vi "main_ctrl.vi"(8 "error in":errorcluster) -> (0 "error out":errorcluster)   [LabVIEW 2011]
uses:
  fg_typedef.ctl
  vision enable.ctl
  vision data.ctl
  singleUseSubstate.ctl
  subStates.ctl
  <vilib>/Rock Robotics/WPI/Solenoid/WPI_SolenoidValue.ctl
  <vilib>/Rock Robotics/WPI/Compressor/WPI_CompressorGetSetRefNum.vi
  <vilib>/Rock Robotics/WPI/Solenoid/WPI_SolenoidGetEnum.vi
  <vilib>/Rock Robotics/WPI/Solenoid/WPI_SolenoidSetEnum.vi
  <vilib>/addons/control/pid/pid.llb/PID Control Input Filter (DBL).vi
  <vilib>/addons/control/pid/NI_PID_pid.lvlib
  <vilib>/Rock Robotics/WPI/RobotDrive/WPI_RobotDriveArcadeDrive_Standard(NoSaturation).vi
panel:
  out "Vision SPI":u32
  out "Vision IPS":dbl
  out "IPS":dbl
  out "SPI":u32
  # "MAIN CONTROL"
  # "holds robot control code - dual parallel state machine"
  # "SPI: milliseconds per iteration\nIPS: iterations per second"
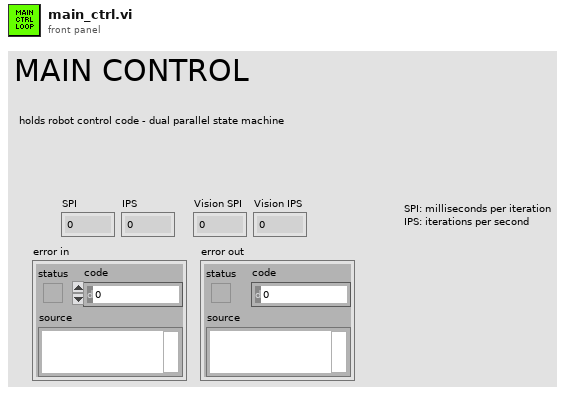
[diagram p1: front panel]
types:
  T1 = typedef "vision data.ctl" = cluster{"x":dbl, "y":dbl, "area":dbl, "width":dbl, "height":dbl}
  T2 = typedef "vision enable.ctl" = enum16{"Enable", "Disable", "Stop"}
  T3 = typedef "fg_typedef.ctl" = enum16{"Get", "Set"}
  T4 = typedef "WPI_CameraDevRef.ctl" = cluster{"Camera Address":string, "CameraStatus":errorcluster, "Acquire Image Notifier":refnum<notifier>}
  T5 = typedef "WPI_CompressorDevRef.ctl" = cluster{"DevStatus":errorcluster, "DigitalInputDevRef":T6, "RelayDevRef":T9}
  T6 = typedef "WPI_DigitalInputDevRef.ctl" = cluster{"DevStatus":errorcluster, "DIO Channel":T7, "Digital Module":T8}
  T7 = typedef "FPGA_DIOChannel.ctl" = enum8{"DIO 1", "DIO 2", "DIO 3", "DIO 4", "DIO 5", "DIO 6", "DIO 7", "DIO 8", "DIO 9", "DIO 10", "DIO 11", "DIO 12", "DIO 13", "DIO 14", "Invalid"}
  T8 = typedef "FPGA_TypedefDigitalModule.ctl" = enum16{"Digital Module 1", "Digital Module 2"}
  T9 = typedef "WPI_RelayDevRef.ctl" = cluster{"DevStatus":errorcluster, "Relay Channel":T10, "Digital Module":T8, "Relay Direction":T11}
  T10 = typedef "FPGA_DIORelayChannel.ctl" = enum8{"Relay 1", "Relay 2", "Relay 3", "Relay 4", "Relay 5", "Relay 6", "Relay 7", "Relay 8", "Invalid"}
  T11 = typedef "WPI_RelayDirection.ctl" = enum16{"Both directions", "Forward only", "Reverse only"}
  T12 = typedef "IMAQ Image.ctl" = refnum<image>
  T13 = typedef "WPI_SolenoidValue.ctl" = enum16{"Off", "On", "Forward", "Reverse"}
  T14 = typedef "singleUseSubstate.ctl" = enum16{"null", "wait", "shift", "shift high", "shift low", "bridge down", "bridge up", "extender in", "extender out", "extender toggle", "end"}
  T15 = typedef "WPI_DriverStationDerivedRobotMode.ctl" = enum16{"Init", "Execute", "Stop"}
  T16 = typedef "WPI_DriverStationRobotMode.ctl" = enum16{"Autonomous Disabled", "Autonomous Enabled", "Teleop Disabled", "Teleop Enabled", "Timeout", "Finish"}
  T17 = typedef "subStates.ctl" = enum16{"null", "wait", "driver control", "auto", "manual override", "autoDrive", "hold position", "rotate", "end"}
  T18 = typedef "WPI_SolenoidDevRef.ctl" = cluster{"DevStatus":errorcluster, "Solenoid Module":T19, "Forward Solenoid Channel":T20, "Reverse Solenoid Channel":T20}
  T19 = typedef "FPGA_TypedefSolenoidModule.ctl" = enum16{"Solenoid Module 1", "Solenoid Module 2"}
  T20 = typedef "WPI_SolenoidChannel.ctl" = enum8{"Solenoid 1", "Solenoid 2", "Solenoid 3", "Solenoid 4", "Solenoid 5", "Solenoid 6", "Solenoid 7", "Solenoid 8", "Invalid"}
  T21 = typedef "WPI_RobotDriveDevRef.ctl" = cluster{"DevStatus":errorcluster, "Motors[]":T22[], "Square Inputs":bool, "Max Output":dbl, "Isochronous":bool}
  T22 = typedef "WPI_MotorControlDeviceRef.ctl" = cluster{"DeviceStatus":errorcluster, "Type":enum16{"PWM", "CAN"}, "PWM":cluster{"Digital Module":T8, "PWM Channel":T23, "DeadBand":T24}, "CAN":cluster{"Device Number":u8, "Control Mode":T25, "Semaphore":T26, "Max Vout":dbl}, "Invert":bool, "TransformRef":T27, "InvTransformRef":T27}
  T23 = typedef "FPGA_DIOPWMChannel.ctl" = enum8{"PWM 1", "PWM 2", "PWM 3", "PWM 4", "PWM 5", "PWM 6", "PWM 7", "PWM 8", "PWM 9", "PWM 10", "Invalid"}
  T24 = typedef "WPI_PWMDeadband.ctl" = cluster{"Name":string, "maxPositivePwm":i32, "minPositivePwm":i32, "centerPwm":i32, "maxNegativePwm":i32, "minNegativePwm":i32, "angularRange":u16}
  T25 = typedef "WPI_CANJaguar_ControlMode.ctl" = enum8{"Percent VBus", "Current", "Speed", "Position", "Voltage"}
  T26 = typedef "Semaphore RefNum" = refnum<k1>
  T27 = typedef "WPI_PWMTransform_ConPane.ctl" = refnum<vi>
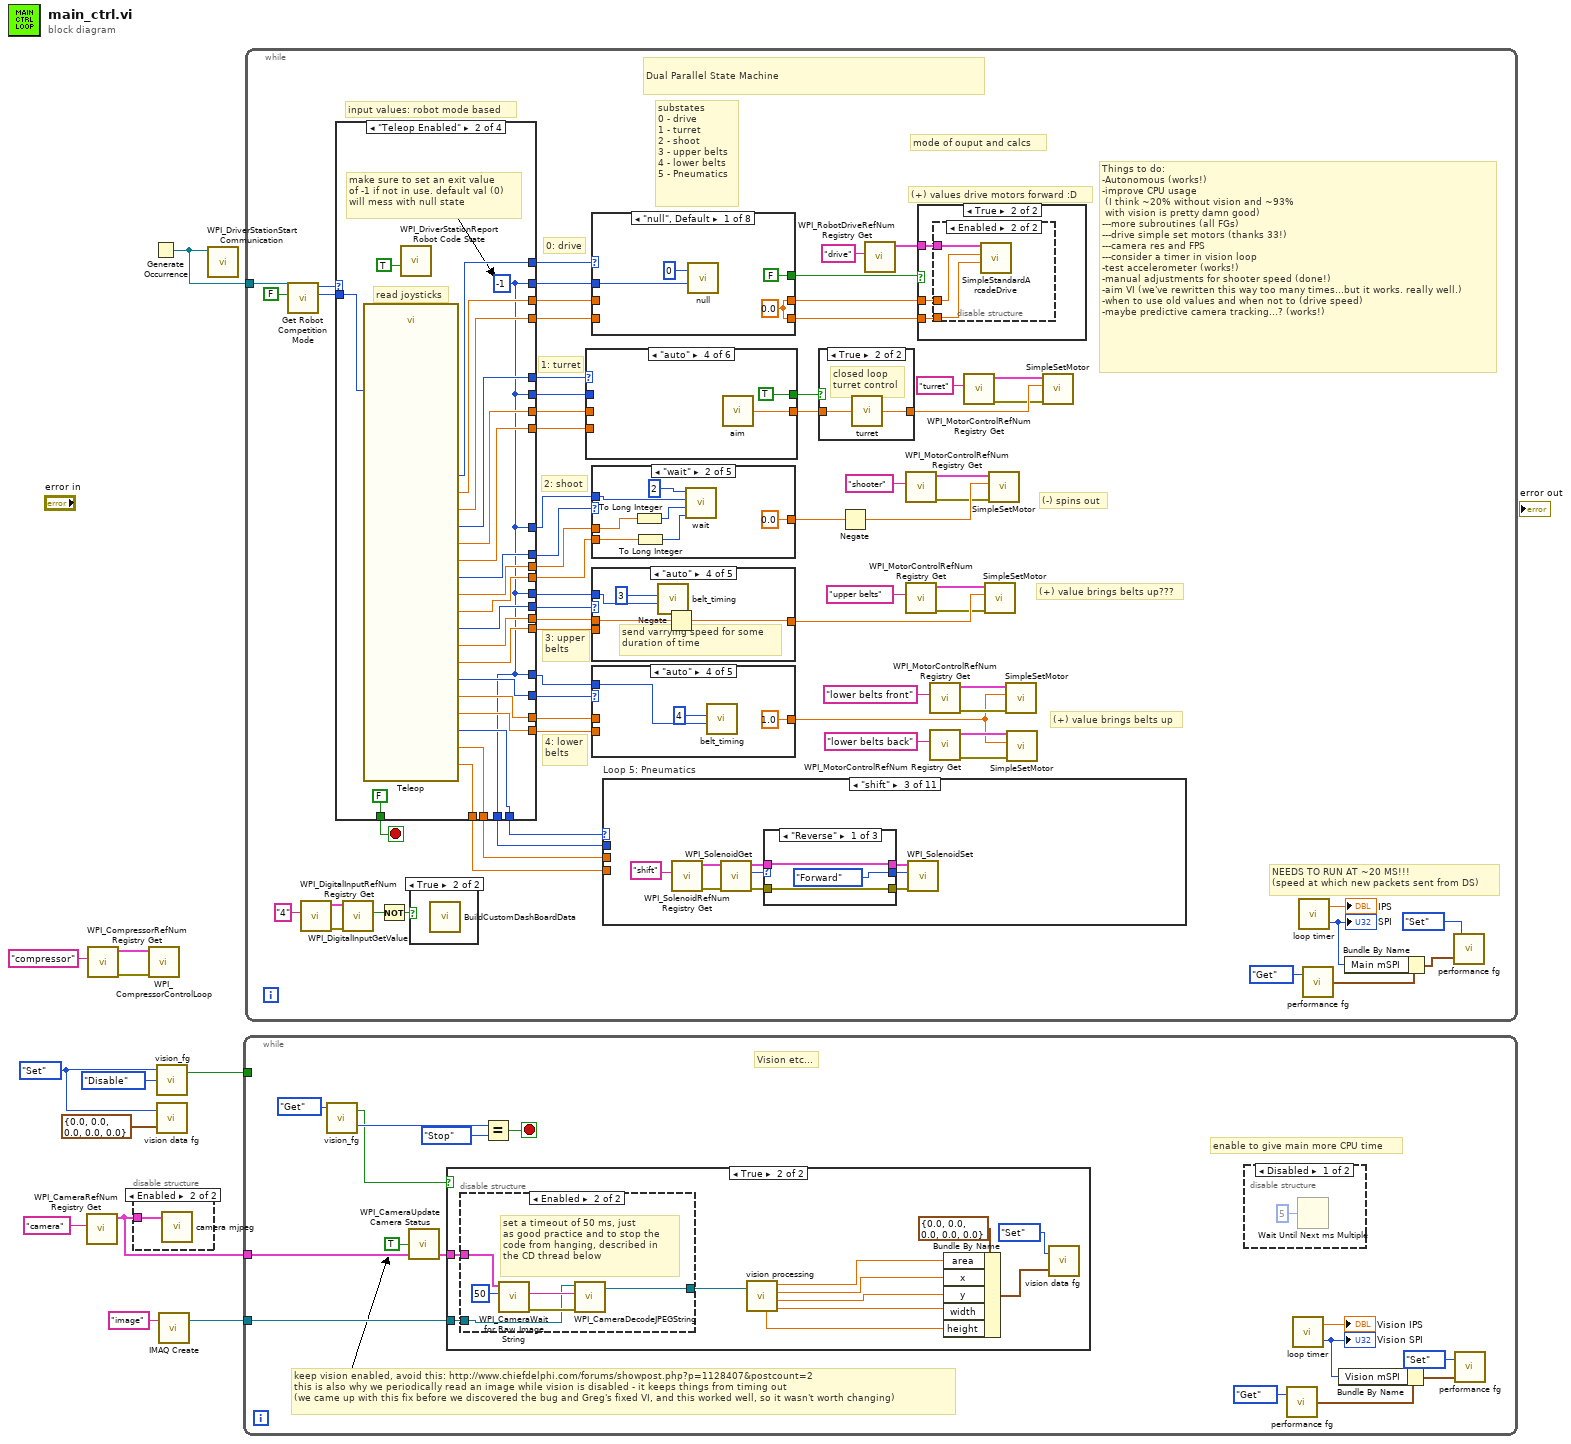
[diagram p0: block diagram]
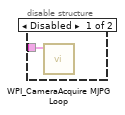
[diagram p2: hidden frame]
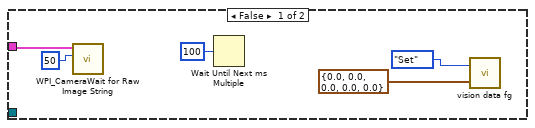
[diagram p4: hidden frame]
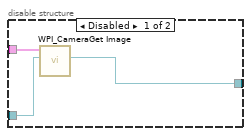
[diagram p5: hidden frame]
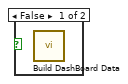
[diagram p6: hidden frame]
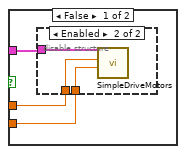
[diagram p8: hidden frame]
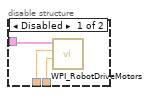
[diagram p9: hidden frame]
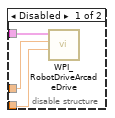
[diagram p10: hidden frame]
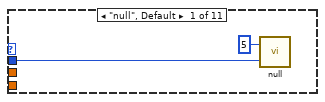
[diagram p11: hidden frame]
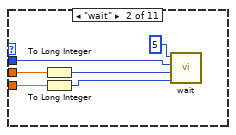
[diagram p12: hidden frame]
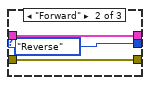
[diagram p13: hidden frame]
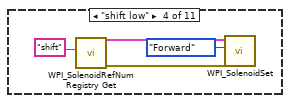
[diagram p15: hidden frame]
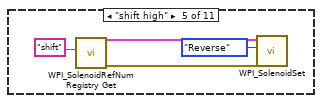
[diagram p16: hidden frame]
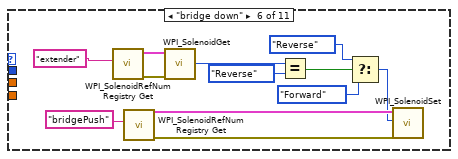
[diagram p17: hidden frame]
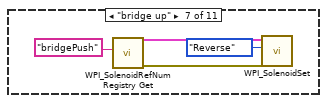
[diagram p18: hidden frame]
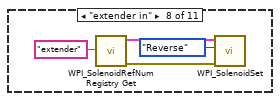
[diagram p19: hidden frame]
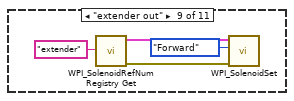
[diagram p20: hidden frame]
diagram:
  w9 = fg_typedef."Set" ("Enum")
  n1 = call <vilib>:"WPI_CameraRefNum Registry Get.vi"("refnum name"="camera") -> ("CameraDevRef"=w2:T4)  [unwired: 9 in, 1 out]
  n2 = call <vilib>:"WPI_CompressorRefNum Registry Get.vi"("refnum name"="compressor") -> ("error out"=w5:errorcluster, "CompressorDevRef"=w6:T5)  [unwired: 9 in]
  n3 = disable-structure shown="Enabled" {
    disable-tunnel: w2 -> [w13 w14]
    frame Disabled {
      n4 = call <vilib>:"WPI_CameraAcquire MJPG Loop.vi"("CameraDevRef"=w13) -> ()  [unwired: 11 in]
    }
    frame Enabled {
      n5 = call "camera mjpeg.vi"("CameraDevRef"=w14) -> ()  [unwired: 11 in]
    }
  }
  n6 = call <vilib>:"WPI_CompressorControlLoop.vi"("error in (no error)"=w5, "CompressorDevRef"=w6) -> ()  [unwired: 10 in]
  n7 = Generate Occurrence() -> (w12:refnum<k4>)
  n8 = call "vision_fg.vi"("Action"=vision_enable."Disable", "Menu"=w9) -> ("Enabled?"=w10:bool)  [unwired: 1 in, 1 out]
  n9 = call "vision data fg.vi"("Input"=T1 {"x"=0.0, "y"=0.0, "area"=0.0, "width"=0.0, "height"=0.0} ("Cluster"), "Menu"=w9) -> ()  [unwired: 1 out]
  n10 = call "IMAQ Create"("Image Name"="image") -> ("New Image"=w11:T12)  [unwired: 4 in, 1 out]
  n11 = call <vilib>:"WPI_DriverStationStart Communication.vi"("occurrence"=w12) -> ()  [unwired: 11 out]
  n12 = while {
    tunnel: w11 -> [w28]
    tunnel: w2 -> [w27]
    tunnel: w10 -> [_]
    stop <- w29 stop-if-true
    # "keep vision enabled, avoid this: http://www.chiefdelphi.com/forums/showpost.php?p=1128407&postcount=2\nthis is also why we periodically read an image while vision is disabled - it keeps things from timing out\n(we came up with this fix before we discovered the bug and Greg's fixed VI, and this worked well, so it wasn't worth changing)"
    # "enable to give main more CPU time"
    # "Vision etc..."
    n13 = call "vision_fg.vi"("Menu"=fg_typedef."Get" ("Enum")) -> ("State Out"=w23:T2, "Enabled?"=w15:bool)  [unwired: 2 in]
    n14 = call <vilib>:"WPI_CameraUpdate Camera Status.vi"("CameraDevRef In"=w27, "Enable Vision"=TRUE) -> ("CameraDevRef Out"=w26:T4)  [unwired: 3 in]
    n15 = case shown="True" w15 {
      tunnel: w28 -> [_ w46]
      tunnel: w26 -> [w33 w45]
      frame False {
        n16 = call <vilib>:"WPI_CameraWait for Raw Image String.vi"("Timeout in ms (-1)"=50, "CameraDevRef"=w33) -> ()  [unwired: 3 in, 7 out]
        n17 = Wait Until Next ms Multiple(millisecond multiple=u32 100) -> ()  [unwired: 1 out]
        n18 = call "vision data fg.vi"("Input"=T1 {"x"=0.0, "y"=0.0, "area"=0.0, "width"=0.0, "height"=0.0} ("Cluster"), "Menu"=fg_typedef."Set" ("Enum")) -> ()  [unwired: 1 out]
      }
      frame True {
        n19 = disable-structure shown="Enabled" {
          disable-tunnel: w46 -> [w49 w51]
          disable-tunnel: w45 -> [w48 w53]
          disable-tunnel: [w47 w50] -> w42
          frame Disabled {
            n20 = call <vilib>:"WPI_CameraGet Image.vi"("Image"=w49, "CameraDevRef"=w48) -> ("Image Out"=w47:T12)  [unwired: 7 in, 2 out]
          }
          frame Enabled {
            # "set a timeout of 50 ms, just\nas good practice and to stop the \ncode from hanging, described in \nthe CD thread below"
            n21 = call <vilib>:"WPI_CameraWait for Raw Image String.vi"("Timeout in ms (-1)"=50, "CameraDevRef"=w53) -> ("error out"=w55:errorcluster, "String"=w54:string)  [unwired: 3 in, 5 out]
            n22 = call <vilib>:"WPI_CameraDecodeJPEGString.vi"("error in"=w55, "Compressed Image"=w54, "Image In"=w51) -> ("Image Out"=w50:T12)  [unwired: 4 out]
          }
        }
        n23 = call "vision processing.vi"("Image In"=w42) -> ("height"=w39:dbl, "area"=w38:dbl, "x"=w37:dbl, "y"=w36:dbl, "width"=w40:dbl)  [unwired: 1 in, 1 out]
        n24 = Bundle By Name(cluster=T1 {"x"=0.0, "y"=0.0, "area"=0.0, "width"=0.0, "height"=0.0} ("Cluster"), "area"=w38, "x"=w37, "y"=w36, "width"=w40, "height"=w39) -> (w41:T1)
        n25 = call "vision data fg.vi"("Input"=w41, "Menu"=fg_typedef."Set" ("Enum")) -> ()  [unwired: 1 out]
      }
    }
    n26 = Equal?(x=w23, y=vision_enable."Stop") -> (x = y?=w29:bool)
    n27 = disable-structure shown="Disabled" {
      frame Disabled {
        n28 = Wait Until Next ms Multiple(millisecond multiple=u32 5) -> ()  [unwired: 1 out]
      }
      frame Enabled {
      }
    }
    n29 = call "performance fg.vi"("Menu"=fg_typedef."Get") -> ("Output"=w18:cluster{"Vision mSPI":u32, "Main mSPI":u32})  [unwired: 1 in]
    n30 = call "loop timer.vi"() -> ("IPS"=→"Vision IPS":dbl, "SPI"=w20:u32)  [unwired: 1 in]
    "Vision SPI" <- w20
    n31 = Bundle By Name(cluster=w18, "Vision mSPI"=w20) -> (w17:cluster{"Vision mSPI":u32, "Main mSPI":u32})
    n32 = call "performance fg.vi"("Input"=w17, "Menu"=fg_typedef."Set") -> ()  [unwired: 1 out]
  }
  n33 = while {
    tunnel: w12 -> [w121]
    stop <- w96 stop-if-true
    # "input values: robot mode based"
    # "Things to do:\n-Autonomous (works!)\n-improve CPU usage\n (I think ~20% without vision and ~93% \n with vision is pretty damn good)\n---more subroutines (all FGs)\n---drive simple set motors (thanks 33!)\n---camera res and FPS\n---consider a timer in vision loop\n-test accelerometer (works!)\n-manual adjustments for shooter speed (done!)\n-aim VI (we've rewritten this way too many times...but it works. really well.)\n-when to use old values and when not to (drive speed)\n-maybe predictive camera tracking...? (works!)"
    # "(-) spins out"
    # "(+) value brings belts up"
    # "(+) values drive motors forward :D"
    # "(+) value brings belts up???"
    # "mode of ouput and calcs"
    # "4: lower\nbelts"
    # "3: upper\nbelts"
    # "2: shoot"
    # "1: turret"
    # "0: drive"
    # "substates\n0 - drive\n1 - turret\n2 - shoot\n3 - upper belts\n4 - lower belts\n5 - Pneumatics"
    # "NEEDS TO RUN AT ~20 MS!!!\n(speed at which new packets sent from DS)"
    # "Dual Parallel State Machine"
    n34 = call "Get Robot Competition Mode.vi"("Finish"=FALSE, "DS Occurrence"=w121) -> ("Call Context"=w110:T15, "Robot Mode"=w120:T16)  [unwired: 6 in, 2 out]
    n35 = call <vilib>:"WPI_DigitalInputRefNum Registry Get.vi"("refnum name"="4") -> ("error out"=w73:errorcluster, "DigitalInputDevRef"=w72:T6)  [unwired: 9 in]
    n36 = case shown="\"Teleop Enabled\"" w120 {
      tunnel: [w342 w364 w368 w380] -> w82
      tunnel: [w341 w361 w368 w380] -> w119
      tunnel: [w340 w345 w366 _] -> w118
      tunnel: [w339 w363 _ _] -> w117
      tunnel: [w338 w362 _ _] -> w116
      tunnel: [w337 w345 w366 _] -> w115
      tunnel: [w336 w359 _ _] -> w114
      tunnel: [w335 w358 _ _] -> w113
      tunnel: w110 -> [w334 w343 _ _]
      tunnel: [w333 w360 w368 w380] -> w107
      tunnel: [w332 w357 _ _] -> w106
      tunnel: [w331 w356 w368 w380] -> w105
      tunnel: [w327 w355 w368 w380] -> w104
      tunnel: [w330 w354 _ _] -> w103
      tunnel: [w326 w353 _ _] -> w102
      tunnel: [w329 w352 _ _] -> w100
      tunnel: [w325 w351 _ _] -> w99
      tunnel: [w324 w346 singleUseSubstate."null" ("SubState 5") singleUseSubstate."end" ("SubState 5")] -> w97
      tunnel: [FALSE FALSE FALSE TRUE] -> w96
      tunnel: [w328 w345 w366 _] -> w83
      tunnel: [w323 w345 w366 _] -> w88
      tunnel: [w322 w345 w366 _] -> w87
      tunnel: [w319 w349 _ _] -> w86
      tunnel: [w318 w348 _ _] -> w85
      tunnel: [w320 w345 w366 _] -> w84
      tunnel: [w317 w347 _ _] -> w80
      frame "Autonomous Enabled" {
        n37 = call "autoSM.vi"("Call Context"=w334) -> ("Loop 2 SubState"=w333:T17, "Loop 2 exit value"=w328:i32, "Loop 2 Value 2"=w317:dbl, "Loop 3 Value 1"=w330:dbl, "Loop 3 Value 2"=w329:dbl, "Loop 2 Value 1"=w332:dbl, "Loop 3 SubState"=w331:T17, "Loop 4 SubState"=w327:T17, "Loop 4 exit value"=w322:i32, "Loop 0 SubState"=w342:T17, "Loop 1 SubState"=w341:T17, "Loop 0 exit value"=w340:i32, "Loop 1 exit value"=w337:i32, "Loop 4 Value 2"=w325:dbl, "Loop 3 exit value"=w323:i32, "Loop 4 Value 1"=w326:dbl, "Pneumatics SubState"=w324:T14, "Loop 0 Value 1"=w339:dbl, "Loop 5 Exit Value"=w320:i32, "Loop 5 Value 2"=w318:dbl, "Loop 0 Value 2"=w338:dbl, "Loop 1 Value 1"=w336:dbl, "Loop 5 Value 1"=w319:dbl, "Loop 1 Value 2"=w335:dbl)  [unwired: 3 in]
        n38 = call <vilib>:"WPI_DriverStationReport Robot Code State.vi"("Autonomous"=TRUE) -> ()  [unwired: 10 in, 1 out]
      }
      frame "Teleop Enabled" {
        w345 = -1 ("Loop 0 exit value")
        # "make sure to set an exit value\nof -1 if not in use. default val (0) \nwill mess with null state"
        # "read joysticks"
        n39 = call "Teleop.vi"("Call Context"=w343) -> ("Loop 5 Value 1"=w349:dbl, "Loop 5 Value 2"=w348:dbl, "Loop 2 Value 2"=w347:dbl, "Loop 2 Value 1"=w357:dbl, "Loop 0 Value 1"=w363:dbl, "Loop 1 Value 2"=w358:dbl, "Loop 4 Value 2"=w351:dbl, "SubState 5"=w346:T14, "Loop 0 Value 2"=w362:dbl, "Loop 1 Value 1"=w359:dbl, "Loop 3 Value 2"=w352:dbl, "Loop 3 Value 1"=w354:dbl, "SubState 0"=w364:T17, "SubState 4"=w355:T17, "SubState 3"=w356:T17, "SubState 1"=w361:T17, "Loop 4 Value 1"=w353:dbl, "SubState 2"=w360:T17)  [unwired: 1 in]
        n40 = call <vilib>:"WPI_DriverStationReport Robot Code State.vi"("TeleOp"=TRUE) -> ()  [unwired: 10 in, 1 out]
      }
      frame "Autonomous Disabled", "Teleop Disabled", "Timeout" {
        w366 = -1 ("Loop 0 exit value")
        w368 = subStates."null" ("SubState 0")
        # "exit value of -1"
        # "set all loops to null"
        # "make sure to disable vision\nwe don't need it here"
        # "robot disabled, timeout"
        n41 = call "vision_fg.vi"("Action"=vision_enable."Disable", "Menu"=fg_typedef."Set") -> ()  [unwired: 1 in, 2 out]
        n42 = call <vilib>:"WPI_DriverStationReport Robot Code State.vi"("Disabled"=TRUE) -> ()  [unwired: 10 in, 1 out]
      }
      frame "Finish" {
        w380 = subStates."end"  # Stop All Loops
        # "stop the while loop"
        # "stop DS comms"
        # "stop compressor"
        # "stop vision loop"
        n43 = call <vilib>:"WPI_DriverStationStop Communication.vi"("StopCommunication"=TRUE) -> ()  [unwired: 10 in, 1 out]
        n44 = call <vilib>:"WPI_CompressorRefNum Registry Get.vi"("refnum name"="compressor") -> ("error out"=w374:errorcluster, "CompressorDevRef"=w373:T5)  [unwired: 9 in]
        n45 = call "vision_fg.vi"("Action"=vision_enable."Stop", "Menu"=fg_typedef."Set") -> ()  [unwired: 1 in, 2 out]
        n46 = call <vilib>:"WPI_CompressorClose.vi"("error in (no error)"=w374, "CompressorDevRef"=w373) -> ()  [unwired: 9 in, 1 out]
      }
    }
    n47 = call <vilib>:"WPI_DigitalInputGetValue.vi"("error in (no error)"=w73, "DigitalInputDevRef"=w72) -> ("Value"=w71:bool)  [unwired: 7 in, 2 out]
    n48 = Not(x=w71) -> (.not. x?=w70:bool)
    n49 = case shown="True" w70 {
      frame False {
        n50 = call "Build DashBoard Data.vi"() -> ()  [unwired: 12 in]
      }
      frame True {
        n51 = call "BuildCustomDashBoardData.vi"() -> ()  [unwired: 12 out]
      }
    }
    n52 = case shown="\"auto\"" w119 {
      tunnel: w115 -> [w255 w263 _ _ _ _]
      tunnel: w114 -> [_ w262 w266 _ _ w273]
      tunnel: w113 -> [_ w260 _ _ _ _]
      tunnel: [0.0 ("Loop 0 Value1") 0.0 ("Loop 1 Value1") w266 w269 0.0 ("Loop 0 Value1") w272] -> w101
      tunnel: [TRUE TRUE TRUE TRUE TRUE FALSE] -> w98
      frame "null", Default {
        n53 = call "null.vi"("Exit Loop ID"=w255, "This Loop ID"=1) -> ()  [unwired: 1 in]
      }
      frame "wait" {
        n54 = To Long Integer(number=w262) -> (32bit integer=w261:i32)
        n55 = To Long Integer(number=w260) -> (32bit integer=w259:i32)
        n56 = call "wait.vi"("State to wait for"=w259, "Waiting Loop ID"=w261, "time (ms)"=w263, "Current Loop ID"=1) -> ()  [unwired: 1 out]
      }
      frame "driver control" {
      }
      frame "auto" {
        n57 = call "aim.vi"() -> ("rate"=w269:dbl)  [unwired: 2 in]
      }
      frame "end" {
      }
      frame "manual override" {
        n58 = expression code="-x/4"(w273) -> (w272:dbl)
      }
    }
    n59 = case shown="\"null\", Default" w82 {
      tunnel: w118 -> [w275 w285 _ _ _ _ _ _]
      tunnel: w117 -> [_ w282 w290 w294 w298 w305 w310 _]
      tunnel: w116 -> [_ w281 w289 w293 w297 w304 w309 _]
      tunnel: [w278 w284 w288 w296 w300 w306 w312 w315] -> w112
      tunnel: [w278 w284 w287 w295 w299 w307 w311 w315] -> w111
      tunnel: [FALSE FALSE TRUE w292 FALSE ("Drive Type") FALSE ("Drive Type") FALSE ("Drive Type") FALSE] -> w109
      frame "null", Default {
        w278 = 0.0 ("Drive Value1")
        n60 = call "null.vi"("Exit Loop ID"=w275, "This Loop ID"=0) -> ()  [unwired: 1 in]
      }
      frame "wait" {
        w284 = 0.0 ("Drive Value1")
        # "wait on timer or parallel state"
        n61 = To Long Integer(number=w282) -> (32bit integer=w280:i32)
        n62 = To Long Integer(number=w281) -> (32bit integer=w279:i32)
        n63 = call "wait.vi"("State to wait for"=w279, "Waiting Loop ID"=w280, "time (ms)"=w285, "Current Loop ID"=0) -> ()  [unwired: 1 out]
      }
      frame "driver control" {
        n64 = Negate(x=w290) -> (-x=w288:dbl)
        n65 = Negate(x=w289) -> (-x=w287:dbl)
      }
      frame "auto" {
        n66 = call "balance.vi"("Joystick X"=w294, "Joystick Y"=w293) -> ("Drive Type"=w292:bool, "left"=w296:dbl, "right"=w295:dbl)
      }
      frame "autoDrive" {
        n67 = call "autoDrive.vi"("Rate"=w297, "Distance to Travel"=w298) -> ("right speed"=w299:dbl, "left speed"=w300:dbl)  [unwired: 1 in, 1 out]
      }
      frame "hold position" {
        n68 = Negate(x=w305) -> (-x=w303:dbl)
        n69 = Negate(x=w304) -> (-x=w302:dbl)
        n70 = call "closed drive.vi"("Y axis value"=w302, "X axis value"=w303) -> ("right"=w307:dbl, "left"=w306:dbl)
      }
      frame "rotate" {
        n71 = call "rotate.vi"("Angle"=w310, "Rate"=w309) -> ("left speed"=w312:dbl, "right speed"=w311:dbl)  [unwired: 1 out]
      }
      frame "end" {
        w315 = 0.0 ("Loop 0 Value1")
      }
    }
    n72 = case shown="\"wait\"" w107 {
      tunnel: w106 -> [_ w245 w249 _ _]
      tunnel: [0.0 ("Loop 2 Value 1") 0.0 ("Loop 2 Value 1") w248 w251 0.0 ("Loop 2 Value 1")] -> w81
      tunnel: w83 -> [w238 w244 _ _ _]
      tunnel: w80 -> [_ w241 _ _ _]
      frame "null", Default {
        n73 = call "null.vi"("Exit Loop ID"=w238, "This Loop ID"=2) -> ()  [unwired: 1 in]
      }
      frame "wait" {
        n74 = To Long Integer(number=w245) -> (32bit integer=w243:i32)
        n75 = To Long Integer(number=w241) -> (32bit integer=w242:i32)
        n76 = call "wait.vi"("State to wait for"=w242, "Waiting Loop ID"=w243, "time (ms)"=w244, "Current Loop ID"=2) -> ()  [unwired: 1 out]
      }
      frame "driver control", "manual override" {
        n77 = expression code="(-x +1) / 2" "can't drive shooter back"(w249) -> (w248:dbl)
      }
      frame "auto" {
        n78 = call "calc shooter speed.vi"() -> ("Speed"=w252:dbl)  [unwired: 1 in]
        n79 = call "battery normalizer.vi"("input"=w252) -> ("output variable"=w250:dbl)
        n80 = call-poly <vilib>:"PID Control Input Filter.vi"("input"=w250) -> ("output"=w251:dbl)  [unwired: 4 in]
      }
      frame "end" {
      }
    }
    n81 = case shown="\"auto\"" w105 {
      tunnel: w103 -> [_ w228 w232 w236 _]
      tunnel: [0.0 ("Loop 2 Value 1") 0.0 ("Loop 2 Value 1") w232 w233 0.0 ("Loop 2 Value 1")] -> w62
      tunnel: w100 -> [_ w225 _ _ _]
      tunnel: w88 -> [w223 w227 _ w235 _]
      frame "null", Default {
        n82 = call "null.vi"("Exit Loop ID"=w223, "This Loop ID"=3) -> ()  [unwired: 1 in]
      }
      frame "wait" {
        n83 = To Long Integer(number=w228) -> (32bit integer=w231:i32)
        n84 = To Long Integer(number=w225) -> (32bit integer=w226:i32)
        n85 = call "wait.vi"("State to wait for"=w226, "Waiting Loop ID"=w231, "time (ms)"=w227, "Current Loop ID"=3) -> ()  [unwired: 1 out]
      }
      frame "driver control" {
      }
      frame "auto" {
        # "send varrying speed for some \nduration of time"
        n86 = call "belt_timing.vi"("time (ms)"=w235, "Loop ID"=3) -> ()  [unwired: 4 in, 1 out]
        n87 = Negate(x=w236) -> (-x=w233:dbl)
      }
      frame "end" {
      }
    }
    n88 = case shown="\"auto\"" w104 {
      tunnel: w102 -> [_ w212 w217 _ _]
      tunnel: [0.0 ("Loop 2 Value 1") 0.0 ("Loop 2 Value 1") w215 1.0 ("Loop 2 Value 1") 0.0 ("Loop 2 Value 1")] -> w57
      tunnel: w99 -> [_ w208 w216 _ _]
      tunnel: w87 -> [w205 w211 _ w218 _]
      frame "null", Default {
        n89 = call "null.vi"("Exit Loop ID"=w205, "This Loop ID"=4) -> ()  [unwired: 1 in]
      }
      frame "wait" {
        n90 = To Long Integer(number=w212) -> (32bit integer=w210:i32)
        n91 = To Long Integer(number=w208) -> (32bit integer=w209:i32)
        n92 = call "wait.vi"("State to wait for"=w209, "Waiting Loop ID"=w210, "time (ms)"=w211, "Current Loop ID"=4) -> ()  [unwired: 1 out]
      }
      frame "driver control" {
        n93 = Subtract(x=w217, y=w216) -> (x-y=w215:dbl)
      }
      frame "auto" {
        n94 = call "belt_timing.vi"("time (ms)"=w218, "Loop ID"=4) -> ()  [unwired: 4 in, 1 out]
      }
      frame "end" {
      }
    }
    n95 = case "Loop 5: Pneumatics" shown="\"shift\"" w97 {
      tunnel: w86 -> [_ w150 _ _ _ _ _ _ _ _ _]
      tunnel: w85 -> [_ w149 _ _ _ _ _ _ _ _ _]
      tunnel: w84 -> [w144 w146 _ _ _ _ _ _ _ _ _]
      frame "null", Default {
        n96 = call "null.vi"("Exit Loop ID"=w144, "This Loop ID"=5) -> ()  [unwired: 1 in]
      }
      frame "wait" {
        n97 = To Long Integer(number=w150) -> (32bit integer=w148:i32)
        n98 = To Long Integer(number=w149) -> (32bit integer=w147:i32)
        n99 = call "wait.vi"("State to wait for"=w147, "Waiting Loop ID"=w148, "time (ms)"=w146, "Current Loop ID"=5) -> ()  [unwired: 1 out]
      }
      frame "shift" {
        n100 = call <vilib>:"WPI_SolenoidRefNum Registry Get.vi"("refnum name"="shift") -> ("error out"=w159:errorcluster, "SolenoidDevRef"=w158:T18)  [unwired: 9 in]
        n101 = call-poly <vilib>:"WPI_SolenoidGet.vi"("error in (no error)"=w159, "SolenoidDevRef"=w158) -> ("error out"=w155:errorcluster, "Value"=w157:T13, "SolenoidDevRef"=w156:T18)  [unwired: 7 in]
        n102 = case shown="\"Reverse\"" w157 {
          selector: w157 -> [_ _ w169]
          tunnel: w156 -> [w162 w166 w168]
          tunnel: w155 -> [w161 w165 w167]
          tunnel: [WPI_SolenoidValue."Forward" ("Value") WPI_SolenoidValue."Reverse" ("Value") w169] -> w154
          tunnel: [w161 w165 w167] -> w153
          tunnel: [w162 w166 w168] -> w152
          frame "Reverse" {
          }
          frame "Forward" {
          }
          frame "On", Default {
          }
        }
        n103 = call-poly <vilib>:"WPI_SolenoidSet.vi"("error in (no error)"=w153, "Value"=w154, "SolenoidDevRef"=w152) -> ()  [unwired: 7 in, 2 out]
      }
      frame "shift low" {
        n104 = call <vilib>:"WPI_SolenoidRefNum Registry Get.vi"("refnum name"="shift") -> ("error out"=w171:errorcluster, "SolenoidDevRef"=w172:T18)  [unwired: 9 in]
        n105 = call-poly <vilib>:"WPI_SolenoidSet.vi"("error in (no error)"=w171, "Value"=WPI_SolenoidValue."Forward", "SolenoidDevRef"=w172) -> ()  [unwired: 7 in, 2 out]
      }
      frame "shift high" {
        n106 = call <vilib>:"WPI_SolenoidRefNum Registry Get.vi"("refnum name"="shift") -> ("error out"=w177:errorcluster, "SolenoidDevRef"=w176:T18)  [unwired: 9 in]
        n107 = call-poly <vilib>:"WPI_SolenoidSet.vi"("error in (no error)"=w177, "Value"=WPI_SolenoidValue."Reverse", "SolenoidDevRef"=w176) -> ()  [unwired: 7 in, 2 out]
      }
      frame "bridge down" {
        n108 = call <vilib>:"WPI_SolenoidRefNum Registry Get.vi"("refnum name"="extender") -> ("error out"=w185:errorcluster, "SolenoidDevRef"=w184:T18)  [unwired: 9 in]
        n109 = call <vilib>:"WPI_SolenoidRefNum Registry Get.vi"("refnum name"="bridgePush") -> ("error out"=w189:errorcluster, "SolenoidDevRef"=w188:T18)  [unwired: 9 in]
        n110 = call-poly <vilib>:"WPI_SolenoidGet.vi"("error in (no error)"=w185, "SolenoidDevRef"=w184) -> ("Value"=w183:T13)  [unwired: 7 in, 2 out]
        n111 = Equal?(x=w183, y=WPI_SolenoidValue."Reverse") -> (x = y?=w181:bool)
        n112 = Select(t=WPI_SolenoidValue."Reverse" ("Value"), s=w181, f=WPI_SolenoidValue."Forward" ("Value")) -> (s? t:f=w178:T13)
        n113 = call-poly <vilib>:"WPI_SolenoidSet.vi"("error in (no error)"=w189, "Value"=w178, "SolenoidDevRef"=w188) -> ()  [unwired: 7 in, 2 out]
      }
      frame "bridge up" {
        n114 = call <vilib>:"WPI_SolenoidRefNum Registry Get.vi"("refnum name"="bridgePush") -> ("error out"=w193:errorcluster, "SolenoidDevRef"=w192:T18)  [unwired: 9 in]
        n115 = call-poly <vilib>:"WPI_SolenoidSet.vi"("error in (no error)"=w193, "Value"=WPI_SolenoidValue."Reverse", "SolenoidDevRef"=w192) -> ()  [unwired: 7 in, 2 out]
      }
      frame "extender in" {
        n116 = call <vilib>:"WPI_SolenoidRefNum Registry Get.vi"("refnum name"="extender") -> ("error out"=w195:errorcluster, "SolenoidDevRef"=w196:T18)  [unwired: 9 in]
        n117 = call-poly <vilib>:"WPI_SolenoidSet.vi"("error in (no error)"=w195, "Value"=WPI_SolenoidValue."Reverse", "SolenoidDevRef"=w196) -> ()  [unwired: 7 in, 2 out]
      }
      frame "extender out" {
        n118 = call <vilib>:"WPI_SolenoidRefNum Registry Get.vi"("refnum name"="extender") -> ("error out"=w198:errorcluster, "SolenoidDevRef"=w199:T18)  [unwired: 9 in]
        n119 = call-poly <vilib>:"WPI_SolenoidSet.vi"("error in (no error)"=w198, "Value"=WPI_SolenoidValue."Forward", "SolenoidDevRef"=w199) -> ()  [unwired: 7 in, 2 out]
      }
      frame "extender toggle" {
      }
      frame "end" {
        n120 = call "states FG.vi"("exit in"=FALSE, "menu (get)"=enum16{"set", "get"}."set", "Loop ID"=5) -> ()  [unwired: 5 in, 4 out]
      }
    }
    n121 = case shown="True" w98 {
      tunnel: [w123 w125] -> w68
      tunnel: w101 -> [w123 w124]
      frame False {
        # "open loop!\nare you sure?"
      }
      frame True {
        # "closed loop\nturret control"
        n122 = call "turret.vi"("rate in (-1 to 1)"=w124) -> ("Output"=w125:dbl)
      }
    }
    n123 = Negate(x=w81) -> (-x=w65:dbl)
    n124 = call <vilib>:"WPI_RobotDriveRefNum Registry Get.vi"("refnum name"="drive") -> ("RobotDriveDevRef"=w89:T21)  [unwired: 9 in, 1 out]
    n125 = call <vilib>:"WPI_MotorControlRefNum Registry Get.vi"("refnum name"="shooter") -> ("error out"=w64:errorcluster, "MotorControlDevRef"=w66:T22)  [unwired: 9 in]
    n126 = call <vilib>:"WPI_MotorControlRefNum Registry Get.vi"("refnum name"="upper belts") -> ("error out"=w61:errorcluster, "MotorControlDevRef"=w63:T22)  [unwired: 9 in]
    n127 = case shown="True" w109 {
      tunnel: w112 -> [w128 w137]
      tunnel: w111 -> [w127 w136]
      tunnel: w89 -> [w126 w135]
      frame False {
        n128 = disable-structure shown="Enabled" {
          disable-tunnel: w128 -> [w131 w133]
          disable-tunnel: w127 -> [w130 w132]
          disable-tunnel: w126 -> [w129 w134]
          frame Disabled {
            n129 = call <vilib>:"WPI_RobotDriveMotors.vi"("RightSpeed"=w130, "LeftSpeed"=w131, "RobotDriveDevRef"=w129) -> ()  [unwired: 1 in, 8 out]
          }
          frame Enabled {
            n130 = call "SimpleDriveMotors.vi"("RightSpeed"=w132, "LeftSpeed"=w133, "RobotDriveDevRef In"=w134) -> ()  [unwired: 7 in, 2 out]
          }
        }
      }
      frame True {
        n131 = disable-structure shown="Enabled" {
          disable-tunnel: w137 -> [w140 w142]
          disable-tunnel: w136 -> [w139 w141]
          disable-tunnel: w135 -> [w138 w143]
          frame Disabled {
            n132 = call-poly <vilib>:"WPI_RobotDriveArcadeDrive.vi"("Y axis value"=w139, "X axis value"=w140, "RobotDriveDevRef"=w138) -> ()  [unwired: 7 in, 2 out]
          }
          frame Enabled {
            n133 = call "SimpleStandardArcadeDrive.vi"("Y axis value"=w141, "X axis value"=w142, "RobotDriveDevRef In"=w143) -> ()  [unwired: 7 in, 2 out]
          }
        }
      }
    }
    n134 = call <vilib>:"WPI_MotorControlRefNum Registry Get.vi"("refnum name"="lower belts front") -> ("error out"=w59:errorcluster, "MotorControlDevRef"=w60:T22)  [unwired: 9 in]
    n135 = call <vilib>:"WPI_MotorControlRefNum Registry Get.vi"("refnum name"="lower belts back") -> ("error out"=w56:errorcluster, "MotorControlDevRef"=w58:T22)  [unwired: 9 in]
    n136 = call <vilib>:"WPI_MotorControlRefNum Registry Get.vi"("refnum name"="turret") -> ("error out"=w67:errorcluster, "MotorControlDevRef"=w69:T22)  [unwired: 9 in]
    n137 = call "SimpleSetMotor.vi"("error in (no error)"=w61, "Output"=w62, "MotorControlDevRef"=w63) -> ()  [unwired: 7 in, 2 out]
    n138 = call "SimpleSetMotor.vi"("error in (no error)"=w64, "Output"=w65, "MotorControlDevRef"=w66) -> ()  [unwired: 7 in, 2 out]
    n139 = call "SimpleSetMotor.vi"("error in (no error)"=w59, "Output"=w57, "MotorControlDevRef"=w60) -> ()  [unwired: 7 in, 2 out]
    n140 = call "SimpleSetMotor.vi"("error in (no error)"=w56, "Output"=w57, "MotorControlDevRef"=w58) -> ()  [unwired: 7 in, 2 out]
    n141 = call "SimpleSetMotor.vi"("error in (no error)"=w67, "Output"=w68, "MotorControlDevRef"=w69) -> ()  [unwired: 7 in, 2 out]
    n142 = call "loop timer.vi"() -> ("IPS"=→"IPS":dbl, "SPI"=w79:u32)  [unwired: 1 in]
    "SPI" <- w79
    n143 = call "performance fg.vi"("Menu"=fg_typedef."Get") -> ("Output"=w76:cluster{"Vision mSPI":u32, "Main mSPI":u32})  [unwired: 1 in]
    n144 = Bundle By Name(cluster=w76, "Main mSPI"=w79) -> (w75:cluster{"Vision mSPI":u32, "Main mSPI":u32})
    n145 = call "performance fg.vi"("Input"=w75, "Menu"=fg_typedef."Set") -> ()  [unwired: 1 out]
  }
